vi "PathPlanner_WPITrajHolPose_New.vi"(9 "HolonomicPose":T1 {"ROTATION"."SIN" format="%13.4f"; "ROTATION"."COS" format="%13.4f"; "ROTATION"."VALUE" format="%13.4f"; "TRANSLATION"."Y" format="%14.3f"; "TRANSLATION"."X" format="%14.3f"}, 11 "TimeSeconds":dbl) -> (3 "WPITrajHolonomicPose":T4 {"HolonomicPose"."ROTATION"."SIN" format="%13.4f"; "HolonomicPose"."ROTATION"."COS" format="%13.4f"; "HolonomicPose"."ROTATION"."VALUE" format="%13.4f"; "HolonomicPose"."TRANSLATION"."Y" format="%14.3f"; "HolonomicPose"."TRANSLATION"."X" format="%14.3f"})   [LabVIEW 2019, in "PathPlanner24.lvlib"]
uses:
  PathPlanner24.lvlib
  TypeDef/PathPlannerWPITrajHolonomicPose.ctl
  <vilib>/Rock Robotics/WPI/ThirdParty/JAS_Junk/TrajLib/TypeDef/POSE2D.ctl
  <vilib>/Rock Robotics/WPI/ThirdParty/JAS_Junk/TrajLib/TypeDef/TRANSLATION2D.ctl
  <vilib>/Rock Robotics/WPI/ThirdParty/JAS_Junk/TrajLib/TypeDef/ROTATION2D.ctl
  <vilib>/Rock Robotics/WPI/ThirdParty/JAS_Junk/TrajLib/Trajectory_Library.lvlib
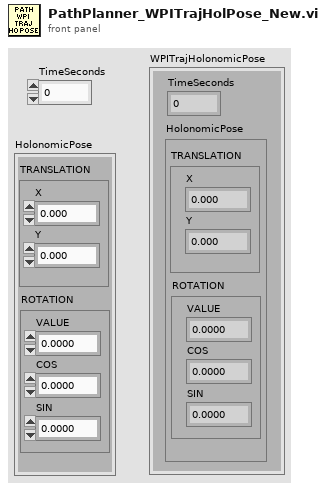
[diagram p1: front panel]
types:
  T1 = typedef "Trajectory_Library.lvlib/POSE2D.ctl" = cluster{"TRANSLATION":T2, "ROTATION":T3}
  T2 = typedef "Trajectory_Library.lvlib/TRANSLATION2D.ctl" = cluster{"X":dbl, "Y":dbl}
  T3 = typedef "Trajectory_Library.lvlib/ROTATION2D.ctl" = cluster{"VALUE":dbl, "COS":dbl, "SIN":dbl}
  T4 = typedef "PathPlanner24.lvlib/PathPlannerWPITrajHolonomicPose.ctl" = cluster{"TimeSeconds":dbl, "HolonomicPose":T1}
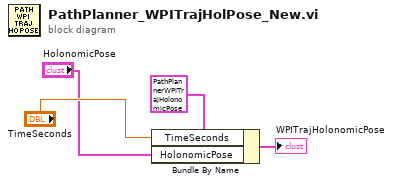
[diagram p0: block diagram]
diagram:
  n1 = Bundle By Name(cluster=T4 {"TimeSeconds"=0.0, "HolonomicPose"={"TRANSLATION"={"X"=0.0, "Y"=0.0}, "ROTATION"={"VALUE"=0.0, "COS"=1.0, "SIN"=0.0}}} ("WPITrajHolonomicPose"), "TimeSeconds"="TimeSeconds", "HolonomicPose"="HolonomicPose") -> (→"WPITrajHolonomicPose":T4)
